vi "Set All.vi"(8 "error in (no error)":errorcluster, 10 "Progress Bar Properties (Default)":T1={"Background Color"=3381759, "Installer Title"="Progress", "Title Color"=0, "Action Text"="", "Text Color"=0, "Slider Value"=0, "Bar Color"=6618880, "Timeout"=10000}) -> (0 "error out":errorcluster)   [LabVIEW 2013, in "Progress Bar.lvlib"]
uses:
  Progress Bar.lvlib
  Controls/Progress Bar Properties.ctl
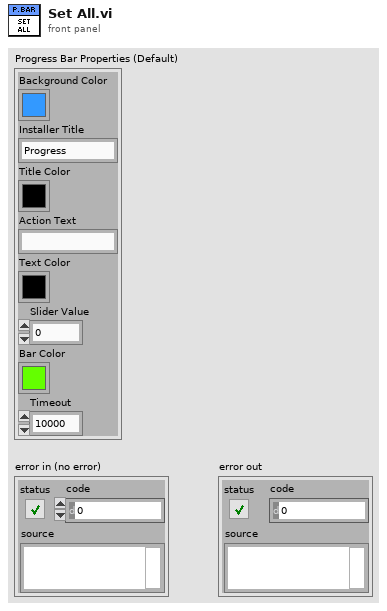
[diagram p1: front panel]
types:
  T1 = typedef "Progress Bar.lvlib/Progress Bar Properties.ctl" = cluster{"Background Color":u32, "Installer Title":string, "Title Color":u32, "Action Text":string, "Text Color":u32, "Slider Value":u8, "Bar Color":u32, "Timeout":i32}
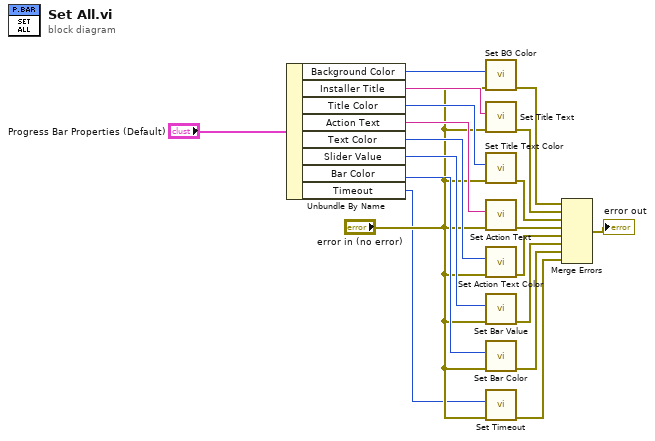
[diagram p0: block diagram]
diagram:
  n1 = Unbundle By Name("Progress Bar Properties (Default)") -> ("Background Color"=w18:u32, "Installer Title"=w17:string, "Title Color"=w16:u32, "Action Text"=w15:string, "Text Color"=w14:u32, "Slider Value"=w13:u8, "Bar Color"=w12:u32, "Timeout"=w1:i32)
  n2 = call "Set BG Color.vi"("error in (no error)"="error in (no error)", "Background Color"=w18) -> ("error out"=w11:errorcluster)  [unwired: 9 in]
  n3 = call "Set Title Text.vi"("error in (no error)"="error in (no error)", "Installer Title"=w17) -> ("error out"=w10:errorcluster)  [unwired: 9 in]
  n4 = call "Set Title Text Color.vi"("error in (no error)"="error in (no error)", "Color Box"=w16) -> ("error out"=w9:errorcluster)  [unwired: 9 in]
  n5 = call "Set Action Text.vi"("error in (no error)"="error in (no error)", "Action Text"=w15) -> ("error out"=w8:errorcluster)  [unwired: 9 in]
  n6 = call "Set Action Text Color.vi"("error in (no error)"="error in (no error)", "Text Color"=w14) -> ("error out"=w7:errorcluster)  [unwired: 9 in]
  n7 = call "Set Bar Value.vi"("error in (no error)"="error in (no error)", "Slider Value"=w13) -> ("error out"=w6:errorcluster)  [unwired: 9 in]
  n8 = call "Set Bar Color.vi"("error in (no error)"="error in (no error)", "Bar Color"=w12) -> ("error out"=w3:errorcluster)  [unwired: 9 in]
  n9 = call "Set Timeout.vi"("error in (no error)"="error in (no error)", "Timeout"=w1) -> ("error out"=w2:errorcluster)  [unwired: 9 in]
  n10 = Merge Errors(w11, w10, w9, w8, w7, w6, w3, w2) -> (→"error out":errorcluster)
